vi "testResult.vi"(11 "Boolean":bool) -> (3 "TestExecution":T1)   [LabVIEW 2015]
uses:
  Typedefs/TestExecution.ctl
  Typedefs/ILCBTTypedefs.lvlib
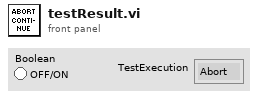
[diagram p1: front panel]
types:
  T1 = typedef "ILCBTTypedefs.lvlib/TestExecution.ctl" = enum16{"Abort", "Continue"}
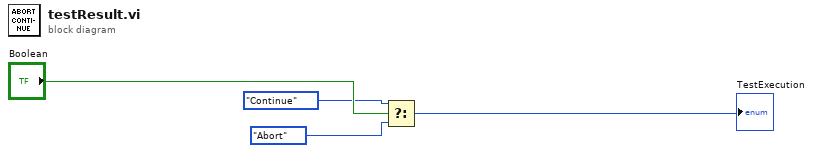
[diagram p0: block diagram]
diagram:
  n1 = Select(t=TestExecution."Continue" ("TestExecution"), s="Boolean", f=TestExecution."Abort" ("TestExecution")) -> (s? t:f=→"TestExecution":T1)
